vi "Prepare Rope Grid List.vi"(1 "Rope Data":T1) -> (0 "Simulated Rope Grid":cluster{string, "H Direction":string}[](array[cluster]))   [LabVIEW 2020, in "AoC 2022.lvlib"]
uses:
  AoC 2022.lvlib
  Rope Data.ctl
  Positions.ctl
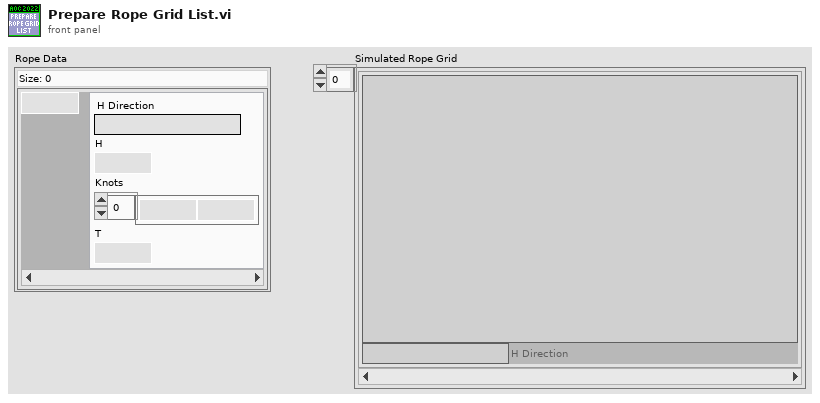
[diagram p1: front panel]
types:
  T1 = typedef "AoC 2022.lvlib/Rope Data.ctl" = map{i32, T2}
  T2 = typedef "AoC 2022.lvlib/Positions.ctl" = cluster{"H Direction":string, "H":cdb, "Knots":cdb[], "T":cdb}
  T3 = cluster{i32, "Rope Grid":cluster{string, "H Direction":string}}
  T4 = cluster{i32, "Rope Grid":cluster{string, "H Direction":string}}[]
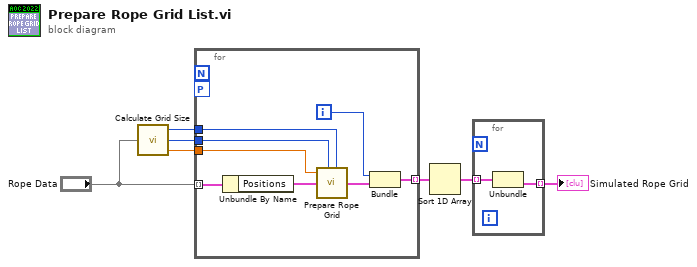
[diagram p0: block diagram]
diagram:
  n1 = call "Calculate Grid Size.vi"("Rope Data"="Rope Data") -> ("Rows"=w5:i32, "Columns"=w6:i32, "Offset"=w1:cdb)
  n2 = for {
    tunnel: w5 -> [w15]
    tunnel: w6 -> [w14]
    tunnel: "Rope Data" -> [w13] mode=indexing
    tunnel: [w11] -> w4 mode=indexing
    workers-P: _ -> [_]
    tunnel: w1 -> [w9]
    i -> [w10]
    n3 = Unbundle By Name(w13) -> ("Positions"=w8:T2)
    n4 = call "Prepare Rope Grid.vi"("Offset"=w9, "Columns"=w14, "Positions"=w8, "Rows"=w15) -> ("Rope Grid"=w12:cluster{string, "H Direction":string})  [unwired: 5 in]
    n5 = Bundle(w10, "Rope Grid"=w12) -> (w11:T3)  [unwired: 1 in]
  }
  n6 = Sort 1D Array(array=w4) -> (sorted array=w3:T4)
  n7 = for {
    tunnel: w3 -> [w17] mode=indexing
    tunnel: [w16] -> w2 mode=indexing
    n8 = Unbundle(w17) -> ("Rope Grid"=w16:cluster{string, "H Direction":string})  [unwired: 1 out]
  }
  "Simulated Rope Grid" <- w2
